vi "Relay basic control.vi"() -> ()   [LabVIEW 2018]
uses:
  <vilib>/DAQmx/read.llb/DAQmx Read (Analog DBL 1Chan 1Samp).vi
  <vilib>/DAQmx/write.llb/DAQmx Write (Analog DBL 1Chan 1Samp).vi
  <vilib>/DAQmx/read.llb/DAQmx Read (Digital 1D Bool NChan 1Samp 1Line).vi
  <vilib>/DAQmx/write.llb/DAQmx Write (Digital 1D Bool NChan 1Samp 1Line).vi
  <vilib>/DAQmx/create/channels.llb/DAQmx Create Channel (DO-Digital Output).vi
  <vilib>/DAQmx/create/channels.llb/DAQmx Create Channel (DI-Digital Input).vi
  <vilib>/DAQmx/create/channels.llb/DAQmx Create Channel (AI-Voltage-Basic).vi
  <vilib>/DAQmx/create/channels.llb/DAQmx Create Channel (AO-Voltage-Basic).vi
  <vilib>/DAQmx/miscellaneous.llb/DAQmx Fill In Error Info.vi
  <vilib>/ptbypt/NI_PtbyPt.lvlib
panel:
  out "Output":dbl format="%.2g"
  out "error 4":errorcluster
  out "Waveform Chart":dbl(graph)
  out "error out 3":errorcluster
  out "Input":dbl format="%0.2f"
  out "error out 2":errorcluster
  in  "data 4":bool
  in  "data 3":bool
  out "error 1":errorcluster
  in  "stop":bool
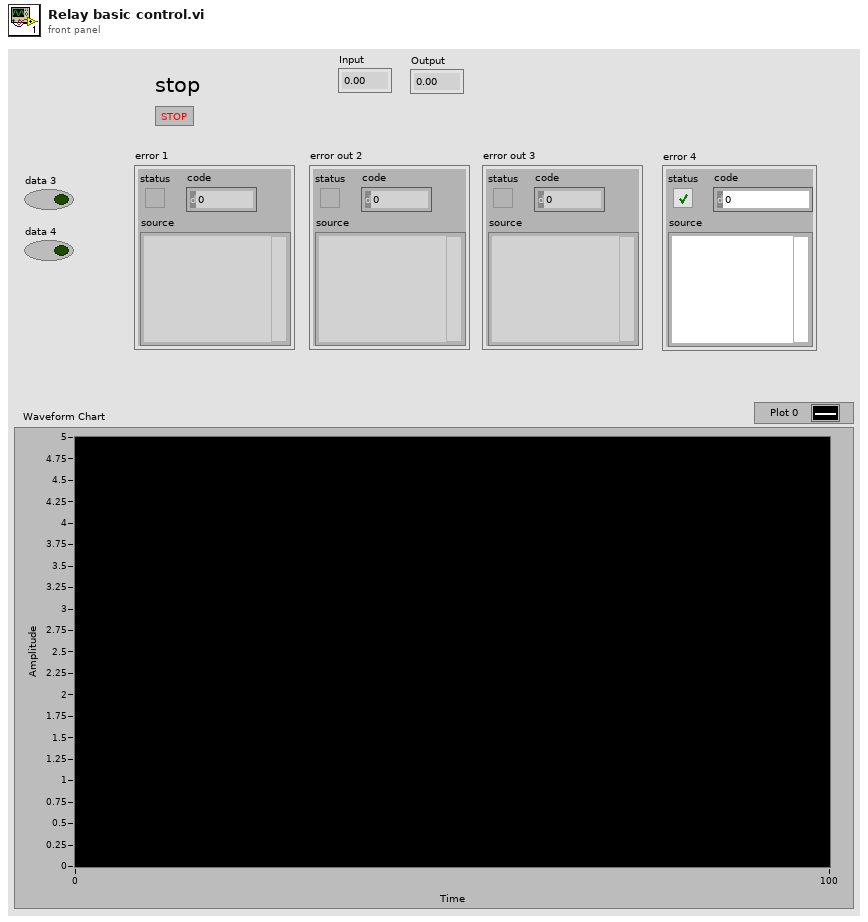
[diagram p1: front panel]
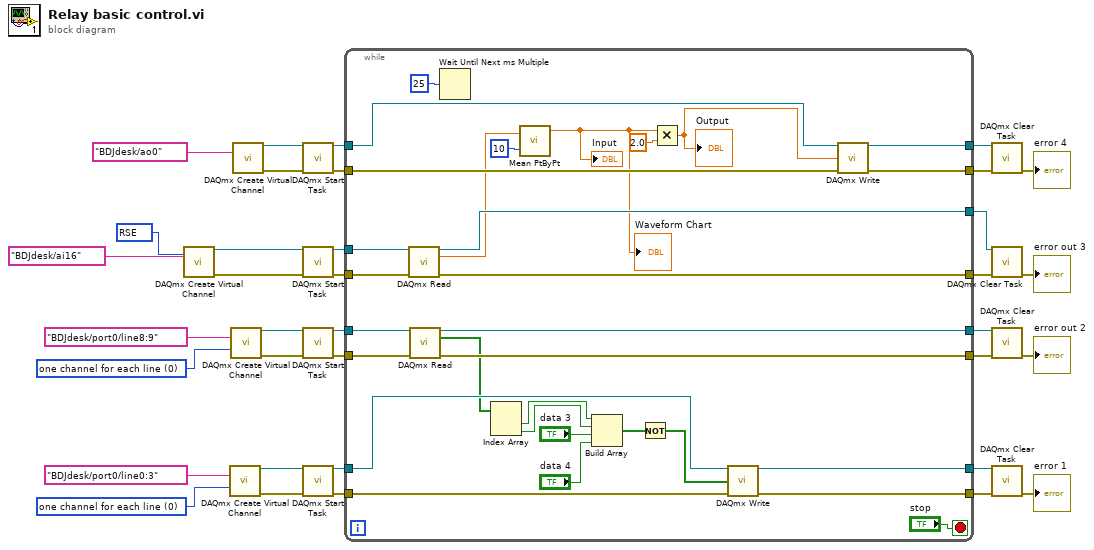
[diagram p0: block diagram]
diagram:
  w16 = 10083 items=["Default"=-1, "RSE"=10083, "NRSE"=10078, "Differential"=10106, "Pseudodifferential"=12529] ("input terminal configuration")
  w25 = 0 items=["one channel for each line", "one channel for all lines"] ("line grouping")
  w27 = 0 items=["one channel for each line", "one channel for all lines"] ("line grouping")
  n1 = call-poly <vilib>:"DAQmx Create Virtual Channel.vi"("input terminal configuration"=w16, "physical channels"=tag "BDJdesk/ai16") -> ("task out"=w15:refnum<k21>, "error out"=w14:errorcluster)  [unwired: 12 in]
  n2 = call-poly <vilib>:"DAQmx Create Virtual Channel.vi"("lines"=tag "BDJdesk/port0/line0:3", "line grouping"=w27) -> ("task out"=w30:refnum<k21>, "error out"=w29:errorcluster)  [unwired: 12 in]
  n3 = call-poly <vilib>:"DAQmx Create Virtual Channel.vi"("lines"=tag "BDJdesk/port0/line8:9", "line grouping"=w25) -> ("task out"=w24:refnum<k21>, "error out"=w21:errorcluster)  [unwired: 12 in]
  n4 = call-poly <vilib>:"DAQmx Create Virtual Channel.vi"("physical channels"=tag "BDJdesk/ao0") -> ("task out"=w5:refnum<k21>, "error out"=w4:errorcluster)  [unwired: 13 in]
  n5 = call <vilib>:"DAQmx Start Task.vi"("task/channels in"=w5, "error in"=w4) -> ("task out"=w3:refnum<k21>, "error out"=w2:errorcluster)  [unwired: 12 in]
  n6 = call <vilib>:"DAQmx Start Task.vi"("task/channels in"=w15, "error in"=w14) -> ("task out"=w13:refnum<k21>, "error out"=w12:errorcluster)  [unwired: 12 in]
  n7 = call <vilib>:"DAQmx Start Task.vi"("task/channels in"=w24, "error in"=w21) -> ("task out"=w23:refnum<k21>, "error out"=w20:errorcluster)  [unwired: 12 in]
  n8 = call <vilib>:"DAQmx Start Task.vi"("task/channels in"=w30, "error in"=w29) -> ("task out"=w35:refnum<k21>, "error out"=w34:errorcluster)  [unwired: 12 in]
  n9 = while {
    tunnel: w35 -> [w65]
    tunnel: [w64] -> w33
    tunnel: w34 -> [w62]
    tunnel: [w61] -> w31
    tunnel: w23 -> [w55]
    tunnel: [w54] -> w22
    tunnel: w20 -> [w53]
    tunnel: [w52] -> w19
    tunnel: w13 -> [w48]
    tunnel: w12 -> [w47]
    tunnel: [w46] -> w11
    tunnel: [w45] -> w10
    tunnel: [w44] -> w7
    tunnel: [w43] -> w6
    tunnel: w3 -> [w42]
    tunnel: w2 -> [w41]
    stop <- "stop" stop-if-true
    n10 = call-poly <vilib>:"DAQmx Read.vi"("task/channels in"=w48, "error in"=w47) -> ("task out"=w46:refnum<k21>, "data"=w38:dbl, "error out"=w45:errorcluster)  [unwired: 11 in]
    n11 = call-poly <vilib>:"DAQmx Read.vi"("task/channels in"=w55, "error in"=w53) -> ("task out"=w54:refnum<k21>, "data"=w51:bool[], "error out"=w52:errorcluster)  [unwired: 11 in]
    n12 = Wait Until Next ms Multiple(millisecond multiple=u32 25) -> ()  [unwired: 1 out]
    n13 = Index Array(array=w51) -> (element #1=w50:bool, element #2=w49:bool)  [unwired: 2 in]
    n14 = call <vilib>:"Mean PtByPt.vi"("x"=w38, "sample length"=10) -> ("mean"=w37:dbl)  [unwired: 2 in, 1 out]
    "Input" <- w37
    "Waveform Chart" <- w37
    n15 = Build Array(w50, w49, "data 3", "data 4") -> (w57:bool[])
    n16 = Not(x=w57) -> (.not. x?=w56:bool[])
    n17 = Multiply(x=w37, y=2.0) -> (x*y=w39:dbl)
    "Output" <- w39
    n18 = call-poly <vilib>:"DAQmx Write.vi"("task/channels in"=w65, "data"=w56, "error in"=w62) -> ("task out"=w64:refnum<k21>, "error out"=w61:errorcluster)  [unwired: 10 in, 1 out]
    n19 = call-poly <vilib>:"DAQmx Write.vi"("task/channels in"=w42, "data"=w39, "error in"=w41) -> ("task out"=w44:refnum<k21>, "error out"=w43:errorcluster)  [unwired: 10 in, 1 out]
  }
  n20 = call <vilib>:"DAQmx Clear Task.vi"("task in"=w7, "error in"=w6) -> ("error out"=→"error 4":errorcluster)  [unwired: 13 in]
  n21 = call <vilib>:"DAQmx Clear Task.vi"("task in"=w11, "error in"=w10) -> ("error out"=→"error out 3":errorcluster)  [unwired: 13 in]
  n22 = call <vilib>:"DAQmx Clear Task.vi"("task in"=w22, "error in"=w19) -> ("error out"=→"error out 2":errorcluster)  [unwired: 13 in]
  n23 = call <vilib>:"DAQmx Clear Task.vi"("task in"=w33, "error in"=w31) -> ("error out"=→"error 1":errorcluster)  [unwired: 13 in]
